vi "FTW-Inbox-Destroy.vi"(0 "FTW Inbox":T1, 11 "error in":errorcluster) -> (15 "error out":errorcluster)   [LabVIEW 2015]
uses:
  core/type/FTW-Type-Actor-Inbox.ctl
panel:
  # "Inputs"
  # "Outputs"
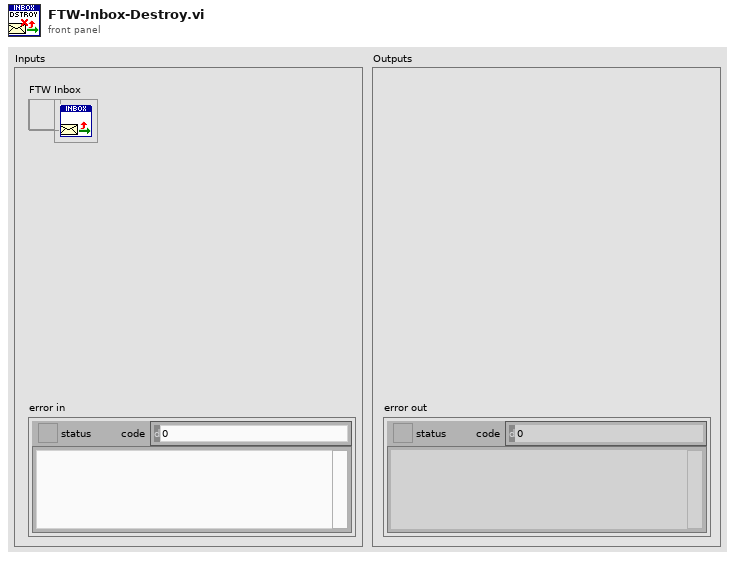
[diagram p1: front panel]
types:
  T1 = typedef "FTW-Type-Actor-Inbox.ctl" = refnum<data-value>
  T2 = cluster{"FTW-CodeGen-Type":enum16{"FTW-Actor-Inbox"}, "Socket":i64}
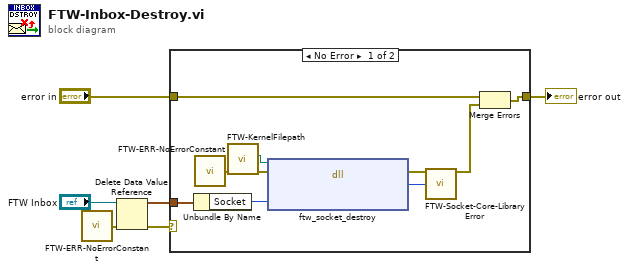
[diagram p0: block diagram]
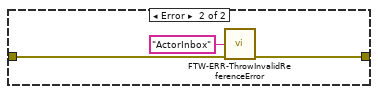
[diagram p2: hidden frame]
diagram:
  n1 = call "FTW-ERR-NoErrorConstant.vi"() -> ("no error"=w1:errorcluster)
  n2 = Delete Data Value Reference(data value reference="FTW Inbox", error in=w1) -> (data value=w3:T2, error out=w2:errorcluster)
  n3 = case shown="No Error" w2 {
    tunnel: [w16 w18] -> w6
    tunnel: "error in" -> [w14 w19]
    tunnel: w3 -> [w12 _]
    frame No Error {
      n4 = Unbundle By Name(w12) -> ("Socket"=w13:i64)
      n5 = call "FTW-ERR-NoErrorConstant.vi"() -> ("no error"=w9:errorcluster)
      n6 = call "FTW-KernelFilepath.vi"("error in"=w9) -> ("error out"=w8:errorcluster, "Library Filepath"=w7:path)  [unwired: 8 in, 1 out]
      n7 = dll-call lib="?" fn="ftw_socket_destroy"(path in=w7, error in=w8, "Socket Handle"=w13) -> (error out=w11:errorcluster, "Return Value"=w10:i64)  [unwired: 2 in, 1 out]
      n8 = call "FTW-Socket-Core-LibraryError.vi"("error in"=w11, "Return Value"=w10) -> ("error out"=w15:errorcluster)  [unwired: 13 in]
      n9 = Merge Errors(w14, w15) -> (w16:errorcluster)
    }
    frame Error {
      n10 = call "FTW-ERR-ThrowInvalidReferenceError.vi"("Reference Type"="ActorInbox", "error in"=w19) -> ("error out"=w18:errorcluster)  [unwired: 13 in]
    }
  }
  "error out" <- w6
